vi "HW_Poll_Tracker_1.x.x.vi"(8 "error in":errorcluster, 11 "VISA resource name in":refnum<visa-resource-name>="ASRL3::INSTR") -> (0 "error out":errorcluster, 1 "Read buffer":string, 2 "Parameters output":T1, 3 "VISA resource name out":refnum<visa-resource-name>)   [LabVIEW 2018, in "HW Interaction.lvlib"]
uses:
  HW Interaction.lvlib
  <vilib>/Utility/error.llb/Error Cluster From Error Code.vi
  <vilib>/ErrorRing/Error Ring.xnode
panel:
  out "Sensors response":string
  out "Port data status":i32
  out "Port data status index":i32
  out "FPS status":i32
  out "Poll records":u32
  out "FPS target index":i32
  out "Matrix mode status":string
  out "Matrix mode index":i32
  out "Coordinate mode status":string
  out "Coordinate mode index":i32
  out "Binary mode status":string
  out "Binary mode index":i32
  out "Array of tokens":string[](array[string])
  out "token index":i32
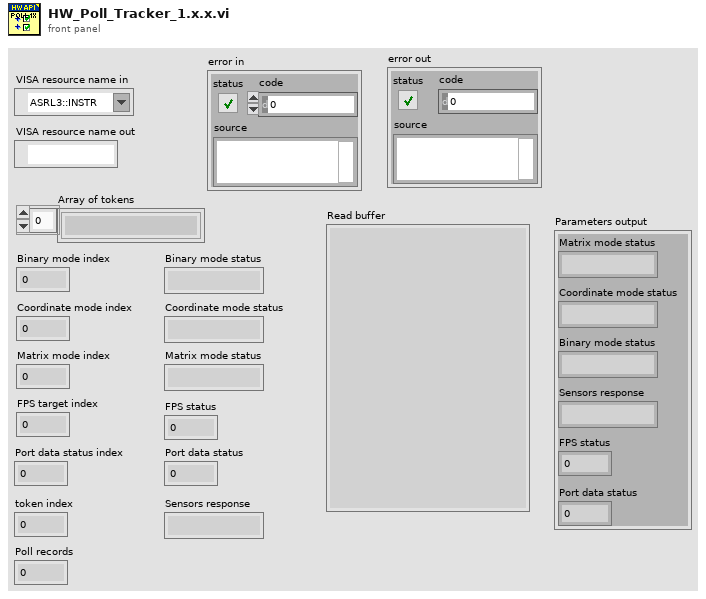
[diagram p1: front panel]
types:
  T1 = cluster{"Matrix mode status":string, "Coordinate mode status":string, "Binary mode status":string, "Sensors response":string, "FPS status":i32, "Port data status":i32}
  T2 = cluster{"token string":string, "token string":string, "token string":string, "trimmed string":string, i32, i32}
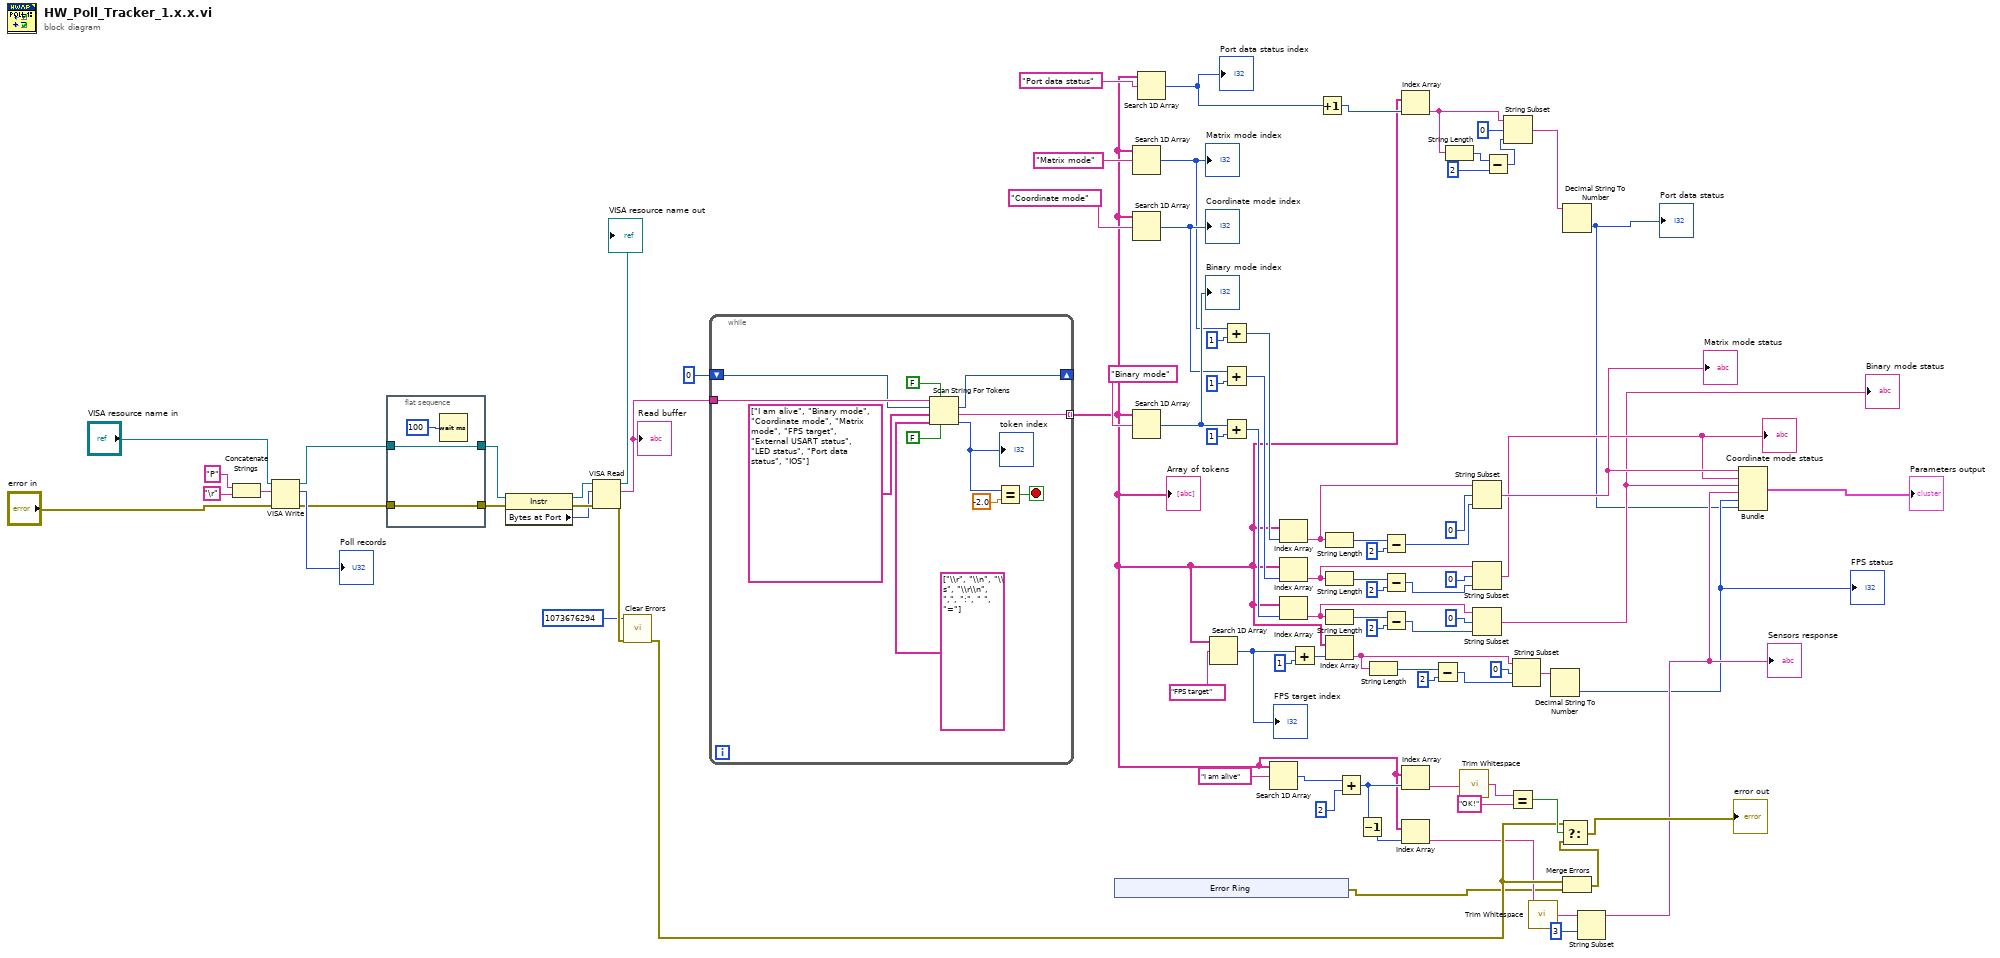
[diagram p0: block diagram]
diagram:
  n1 = Concatenate Strings("P" ("write buffer"), "\r") -> (w86:string)
  n2 = VISA Write(VISA resource name="VISA resource name in", write buffer=w86, error in (no error)="error in") -> (VISA resource name out=w62:refnum<visa-resource-name>, return count=→"Poll records":u32, error out=w60:errorcluster)
  n3 = flat-sequence {
    tunnel: [w90] -> w63
    tunnel: w62 -> [w90]
    tunnel: [w89] -> w61
    tunnel: w60 -> [w89]
    frame #0 {
      n4 = Wait (ms)(milliseconds to wait=u32 100) -> ()  [unwired: 1 out]
    }
  }
  n5 = property class="Instr"(reference=w63, error in=w61) -> (reference out=w84:refnum<visa-resource-name>, error out=w83:errorcluster, "Bytes at Port"=w82:u32)
  n6 = VISA Read(VISA resource name=w84, byte count=w82, error in (no error)=w83) -> (VISA resource name out=→"VISA resource name out":refnum<visa-resource-name>, read buffer=w81:string, error out=w19:errorcluster)  [unwired: 1 out]
  "Read buffer" <- w81
  n7 = call <vilib>:"Clear Errors.vi"("error in (no error)"=w19, "specific error code to clear (0: all)"=1073676294) -> ("error out"=w18:errorcluster)  [unwired: 4 in, 1 out]
  n8 = while {
    tunnel: w81 -> [w102]
    tunnel: [w94] -> w15 mode=indexing
    shift-right: [w93] -> _
    shift-left: 0 ("offset past token") -> [w92]
    stop <- w100 stop-if-true
    n9 = Scan String For Tokens(4:FALSE ("use cached delim/oper data? (F)"), 5:FALSE ("allow empty tokens? (F)"), 6:string[] ["\\r", "\\n", "\\s", "\\r\\n", ",", ":", " ", "="] ("delimiters"), 7:string[] ["I am alive", "Binary mode", "Coordinate mode", "Matrix mode", "FPS target", "External USART status", "LED status", "Port data status", "IOS"] ("Tokens"), 8:w92, 9:w102) -> (0:w98:i32, 1:w94:string, 2:w93:i32)  [unwired: 1 out]
    "token index" <- w98
    n10 = Equal?(x=w98, y=-2.0) -> (x = y?=w100:bool)
  }
  "Array of tokens" <- w15
  n11 = xnode "Error Ring"() -> ("error out"=w1:errorcluster)
  n12 = Search 1D Array(1D array=w15, element="Matrix mode") -> (index of element=w70:i32)  [unwired: 1 in]
  "Matrix mode index" <- w70
  n13 = Search 1D Array(1D array=w15, element="Coordinate mode") -> (index of element=w74:i32)  [unwired: 1 in]
  "Coordinate mode index" <- w74
  n14 = Search 1D Array(1D array=w15, element="Binary mode") -> (index of element=w78:i32)  [unwired: 1 in]
  "Binary mode index" <- w78
  n15 = Search 1D Array(1D array=w15, element="Port data status") -> (index of element=w36:i32)  [unwired: 1 in]
  "Port data status index" <- w36
  n16 = Search 1D Array(1D array=w15, element="FPS target") -> (index of element=w66:i32)  [unwired: 1 in]
  "FPS target index" <- w66
  n17 = Add(x=w70, y=1) -> (x+y=w71:i32)
  n18 = Add(x=w74, y=1) -> (x+y=w75:i32)
  n19 = Add(x=w78, y=1) -> (x+y=w79:i32)
  n20 = Search 1D Array(1D array=w15, element="I am alive") -> (index of element=w27:i32)  [unwired: 1 in]
  n21 = Index Array(array=w15, index=w71) -> (element=w40:string)
  n22 = Index Array(array=w15, index=w75) -> (element=w38:string)
  n23 = Index Array(array=w15, index=w79) -> (element=w57:string)
  n24 = Add(x=w66, y=1) -> (x+y=w67:i32)
  n25 = Increment(x=w36) -> (x+1=w35:i32)
  n26 = String Length(string=w40) -> (length=w52:i32)
  n27 = String Length(string=w38) -> (length=w43:i32)
  n28 = String Length(string=w57) -> (length=w56:i32)
  n29 = Index Array(array=w15, index=w67) -> (element=w39:string)
  n30 = Add(x=w27, y=2) -> (x+y=w16:i32)
  n31 = Decrement(x=w16) -> (x-1=w14:i32)
  n32 = String Length(string=w39) -> (length=w48:i32)
  n33 = Subtract(x=w52, y=2) -> (x-y=w50:i32)
  n34 = Subtract(x=w43, y=2) -> (x-y=w41:i32)
  n35 = Subtract(x=w56, y=2) -> (x-y=w54:i32)
  n36 = Index Array(array=w15, index=w35) -> (element=w34:string)
  n37 = Index Array(array=w15, index=w16) -> (element=w25:string)
  n38 = Index Array(array=w15, index=w14) -> (element=w13:string)
  n39 = Subtract(x=w48, y=2) -> (x-y=w46:i32)
  n40 = String Length(string=w34) -> (length=w33:i32)
  n41 = call <vilib>:"Trim Whitespace.vi"("string"=w25) -> ("trimmed string"=w24:string)  [unwired: 1 in]
  n42 = String Subset(string=w40, offset (0)=0, length (rest)=w50) -> (substring=w10:string)
  "Matrix mode status" <- w10
  n43 = String Subset(string=w38, offset (0)=0, length (rest)=w41) -> (substring=w9:string)
  "Coordinate mode status" <- w9
  n44 = String Subset(string=w57, offset (0)=0, length (rest)=w54) -> (substring=w8:string)
  "Binary mode status" <- w8
  n45 = Subtract(x=w33, y=2) -> (x-y=w31:i32)
  n46 = String Subset(string=w34, offset (0)=0, length (rest)=w31) -> (substring=w29:string)
  n47 = Equal?(x=w24, y="OK!") -> (x = y?=w22:bool)
  n48 = String Subset(string=w39, offset (0)=0, length (rest)=w46) -> (substring=w45:string)
  n49 = call <vilib>:"Trim Whitespace.vi"("string"=w13) -> ("trimmed string"=w12:string)  [unwired: 1 in]
  n50 = Decimal String To Number(string=w45) -> (number=w6:i32)  [unwired: 2 in, 1 out]
  "FPS status" <- w6
  n51 = Decimal String To Number(string=w29) -> (number=w5:i32)  [unwired: 2 in, 1 out]
  "Port data status" <- w5
  n52 = Merge Errors(w18, w1) -> (w20:errorcluster)
  n53 = Select(t=w18, s=w22, f=w20) -> (s? t:f=→"error out":errorcluster)
  n54 = String Subset(string=w12, offset (0)=3) -> (substring=w7:string)  [unwired: 1 in]
  "Sensors response" <- w7
  n55 = Bundle("token string"=w10, "token string"=w9, "token string"=w8, "trimmed string"=w7, w6, w5) -> (→"Parameters output":T2)  [unwired: 1 in]
